vi "Start Remote Data.vi"(8 "error in (no error)":errorcluster, 11 "Vecto in":refnum<class "Vecto.lvclass">) -> (0 "error out":errorcluster, 3 "Vecto out":refnum<class "Vecto.lvclass">)   [LabVIEW 2020, in "Vecto.lvlib" / "Vecto.lvclass"]
uses:
  Vecto.lvclass
  Vecto.lvclass/Vecto.ctl
  RemoteDataService/RemoteDataService.lvclass
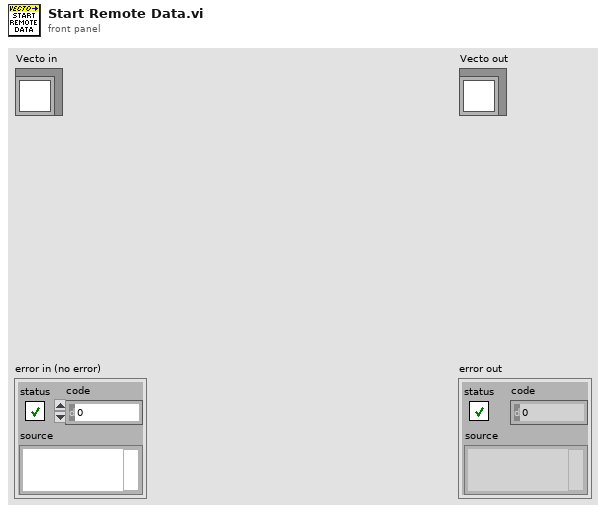
[diagram p1: front panel]
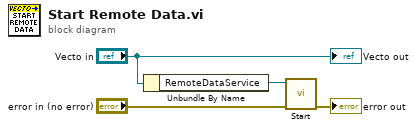
[diagram p0: block diagram]
diagram:
  n1 = Unbundle By Name("Vecto in") -> ("RemoteDataService"=w3:refnum<class "RemoteDataService.lvclass">)
  n2 = call "Start.vi"("error in (no error)"="error in (no error)", "RemoteDataService in"=w3) -> ("error out"=→"error out":errorcluster)  [unwired: 8 in, 1 out]
  "Vecto out" <- "Vecto in"
